vi "LEIN slave detail information.vi"(11 "error in (no error)":errorcluster) -> (15 "error out":errorcluster)   [LabVIEW 2011]
uses:
  LEINmaster/Defenitions/LEIN ID Stat15 and Address.ctl
  LEINmaster/Defenitions/LEIN STAT 15 Id system cluster v2.ctl
  emi Lib/Basic/0 - General/App/Version/Private/_emi_Version Holder.vi
panel:
  out "Pressure node 2":T1 {"LEIN address" format="%.0x"; "ID"."LEIN impl. code" format="%02x"; "ID"."Serial number" format="%04.0f"; "ID"."HW ID" format="%02x"; "ID"."FW ID" format="%02x"; "ID"."HW REV" format="%02x"; "ID"."FW REV" format="%02x"}
  out "Pressure node 1":T1 {"LEIN address" format="%.0x"; "ID"."LEIN impl. code" format="%02x"; "ID"."Serial number" format="%04.0f"; "ID"."HW ID" format="%02x"; "ID"."FW ID" format="%02x"; "ID"."HW REV" format="%02x"; "ID"."FW REV" format="%02x"}
  out "Solenoid":T1 {"LEIN address" format="%.0x"; "ID"."LEIN impl. code" format="%02x"; "ID"."Serial number" format="%04.0f"; "ID"."HW ID" format="%02x"; "ID"."FW ID" format="%02x"; "ID"."HW REV" format="%02x"; "ID"."FW REV" format="%02x"}
  out "Tool controller":T1 {"LEIN address" format="%.0x"; "ID"."LEIN impl. code" format="%02x"; "ID"."Serial number" format="%04.0f"; "ID"."HW ID" format="%02x"; "ID"."FW ID" format="%02x"; "ID"."HW REV" format="%02x"; "ID"."FW REV" format="%02x"}
  in  "Help":bool
  out "OK":bool
  in  "OK btn":bool
  # "Tab header s can be changed as wanted\n\nCustom can be used for completly ccutom behavior,\nmust then highjack  an other hidden page, for settings"
  # "Add custom behavior taht cvan not be replicated by a simple cluster with valisdity checking"
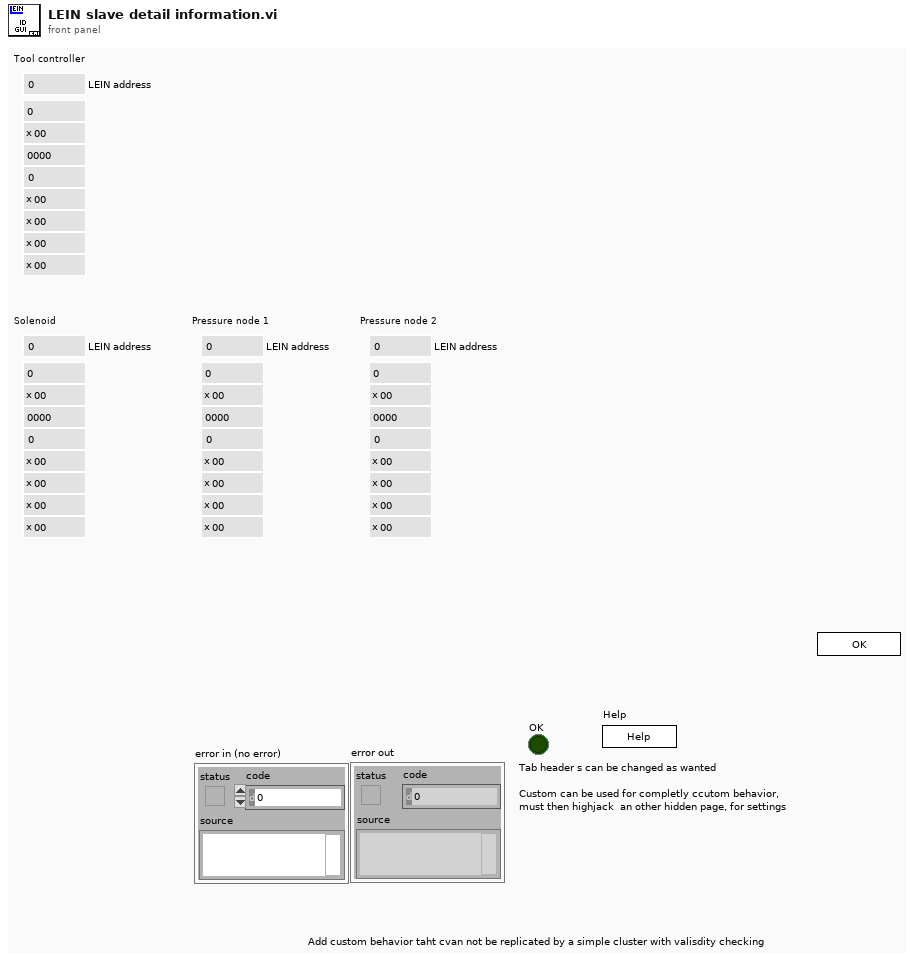
[diagram p1: front panel]
types:
  T1 = typedef "LEIN ID Stat15 and Address.ctl" = cluster{"LEIN address":u8, "ID":T2}
  T2 = typedef "LEIN STAT 15 Id system cluster v2.ctl" = cluster{"LEIN version":u8, "LEIN impl. code":u8, "Serial number":u16, "Project":u16, "HW ID":u8, "FW ID":u8, "HW REV":u8, "FW REV":u8}
  T3 = typedef "emi_Version Info.ctl" = cluster{"Name":string, "Major":i16, "Minor":i16, "Fix":i16, "Build":i32, "Type":enum16{"Alfa", "Beta", "Stable"}, "Dev":bool, "Version Name":string, "Date":timestamp}
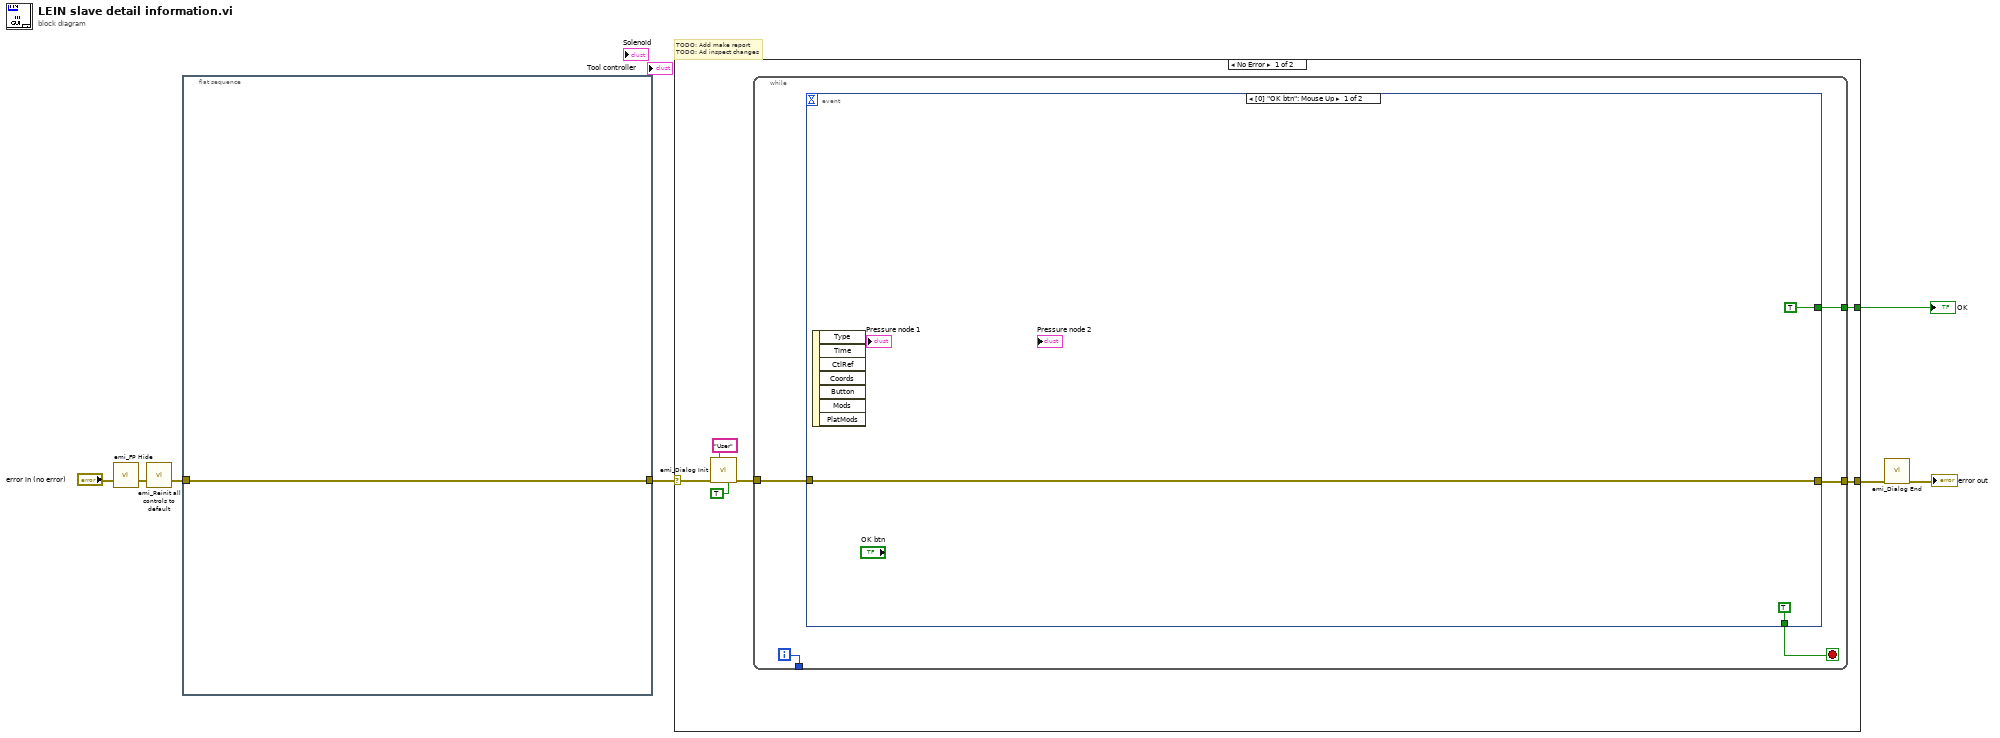
[diagram p0: block diagram]
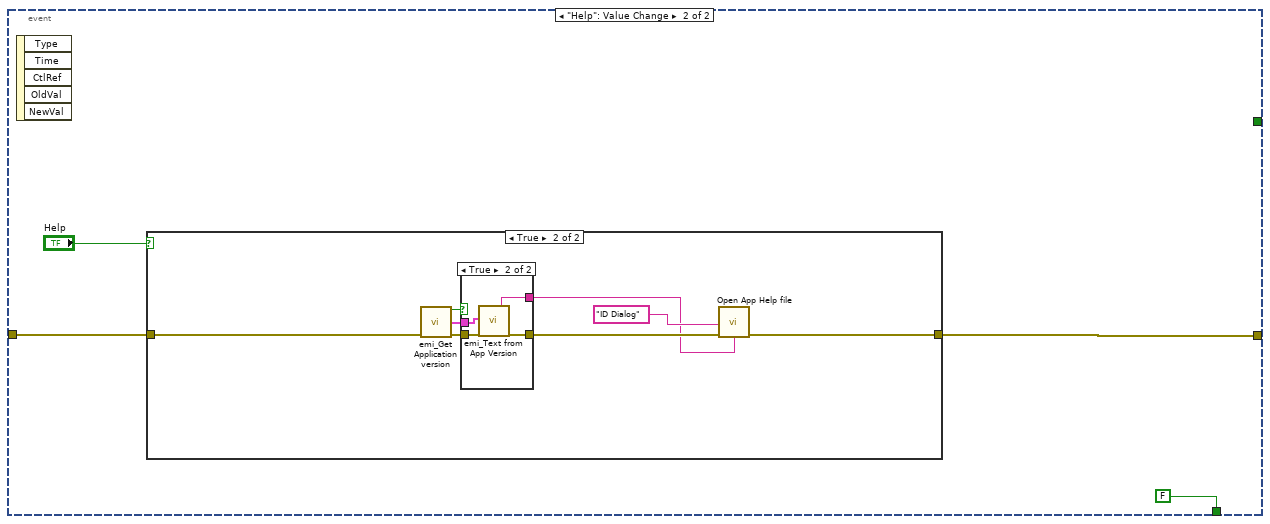
[diagram p2: hidden frame]
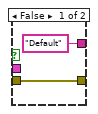
[diagram p4: hidden frame]
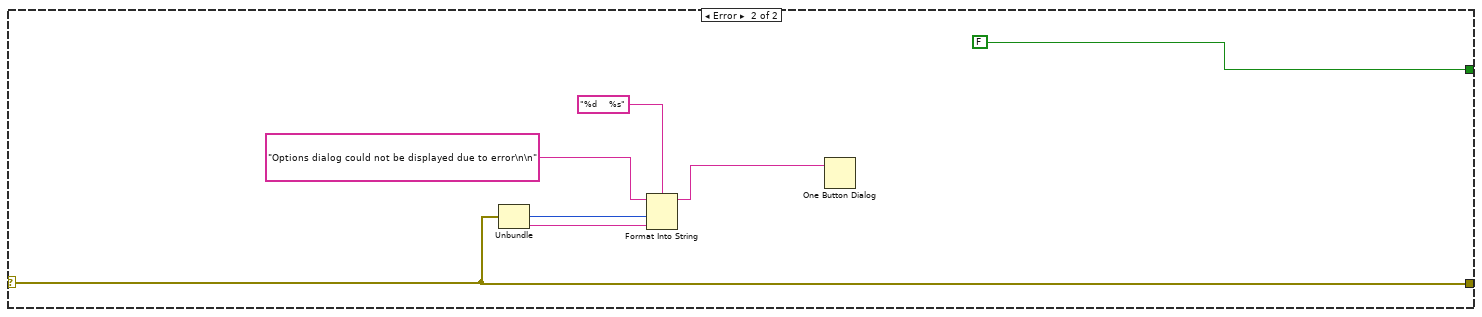
[diagram p5: hidden frame]
diagram:
  # "TODO: Add make report\nTODO: Ad inspect changes"
  n1 = call "emi_FP Hide.vi"("error in (no error)"="error in (no error)") -> ("error out"=w3:errorcluster)  [unwired: 13 in, 1 out]
  n2 = call "emi_Reinit all controls to default.vi"("error in (no error)"=w3) -> ("error out"=w1:errorcluster)  [unwired: 13 in, 1 out]
  n3 = flat-sequence {
    tunnel: w1 -> [w8]
    tunnel: [w8] -> w2
    frame #0 {
    }
  }
  n4 = case shown="No Error" w2 {
    selector: w2 -> [w9 w47]
    tunnel: [w14 FALSE] -> w6
    tunnel: [w13 w47] -> w5
    frame No Error {
      n5 = call "emi_Dialog Init.vi"("Header String(\"\")"="User" ("Header String(\"\")"), "error in"=w9, "Modal(T)"=TRUE) -> ("error out"=w12:errorcluster)  [unwired: 12 in]
      n6 = while {
        tunnel: [w19] -> _
        tunnel: w12 -> [w17]
        tunnel: [w16] -> w13
        tunnel: [w15] -> w14
        i -> [w19]
        stop <- w18 stop-if-true
        n7 = event shown="[0] \"OK btn\": Mouse Up" {
          selector: _ -> [_ _]
          dyn-events: _ -> [_ _]
          timeout: _ -> [_ _]
          tunnel: [TRUE FALSE] -> w18
          tunnel: w17 -> [w20 w24]
          tunnel: [w20 w25] -> w16
          tunnel: [TRUE _] -> w15
          event "OK btn": Mouse Up {
            n8 = event-data() -> ()  [unwired: 1 in, 7 out]
          }
          event "Help": Value Change {
            n9 = event-data() -> ()  [unwired: 1 in, 5 out]
            n10 = case shown="True" "Help" {
              tunnel: [w27 w28] -> w25
              tunnel: w24 -> [w27 w29]
              frame False {
              }
              frame True {
                n11 = call "emi_Get Application version.vi"("error in (no error)"=w29) -> ("Version has been set"=w33:bool, "Version Info out"=w32:T3, "error out"=w31:errorcluster)  [unwired: 12 in]
                n12 = case shown="True" w33 {
                  tunnel: w31 -> [w37 w41]
                  tunnel: w32 -> [_ w40]
                  tunnel: [w37 w39] -> w35
                  tunnel: ["Default" w38] -> w30
                  frame False {
                  }
                  frame True {
                    n13 = call "emi_Text from App Version.vi"("Version Info"=w40, "error in (no error)"=w41) -> ("Name"=w38:string, "error out"=w39:errorcluster)  [unwired: 8 in, 8 out]
                  }
                }
                n14 = call "Open App Help file.vi"("Help Tag (\"\")"="ID Dialog" ("Help Tag (\"\")"), "error In"=w35, "file name(\"App\".chm)"=w30) -> ("error out"=w28:errorcluster)  [unwired: 12 in]
              }
            }
          }
        }
      }
    }
    frame Error {
      n15 = Unbundle(w47) -> ("code"=w44:i32, "source"=w43:string)  [unwired: 1 out]
      n16 = Format Into String(format string="%d    %s", initial string="Options dialog could not be displayed due to error\n\n" ("message"), w44, w43) -> (resulting string=w45:string)  [unwired: 1 in, 1 out]
      n17 = One Button Dialog(message=w45) -> ()  [unwired: 1 in, 1 out]
    }
  }
  "OK" <- w6
  n18 = call "emi_Dialog End.vi"("error in"=w5) -> ("error out"=→"error out":errorcluster)  [unwired: 14 in]
